vi "test Find and Initialize SLSC Switch CD.vi"(8 "error in (no error)":errorcluster, 11 "TestCase in":refnum<class "SLSC Switch Scripting Unit Tests.lvclass">) -> (0 "error out":errorcluster, 3 "TestCase out":refnum<class "SLSC Switch Scripting Unit Tests.lvclass">)   [LabVIEW 2017, in "SLSC Switch Scripting Unit Tests.lvclass"]
uses:
  SLSC Switch Scripting Unit Tests.lvclass
  C:/Program Files (x86)/National Instruments/LabVIEW 2017/vi.lib/addons/_JKI Toolkits/VI Tester/TestCase.llb/TestCase.lvclass
  <vilib>/addons/_JKI Toolkits/VI Tester/TestCase.llb/TestCase.lvclass
panel:
  in  "Save?":bool
  out "Output Filename":string
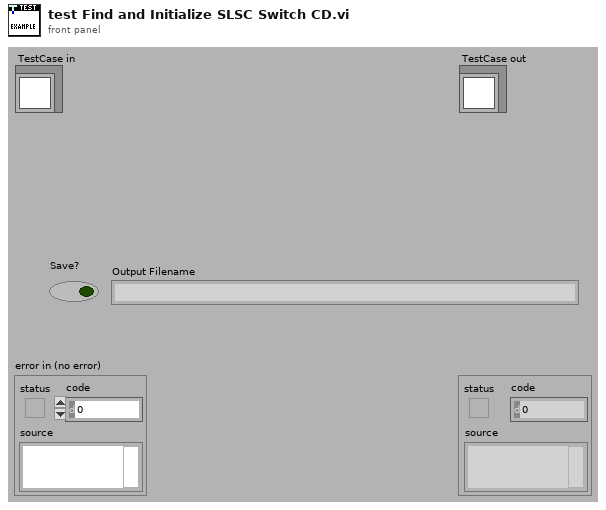
[diagram p1: front panel]
types:
  T1 = typedef "Custom Device API.lvlib/Custom Device Item Ref.ctl" = u64
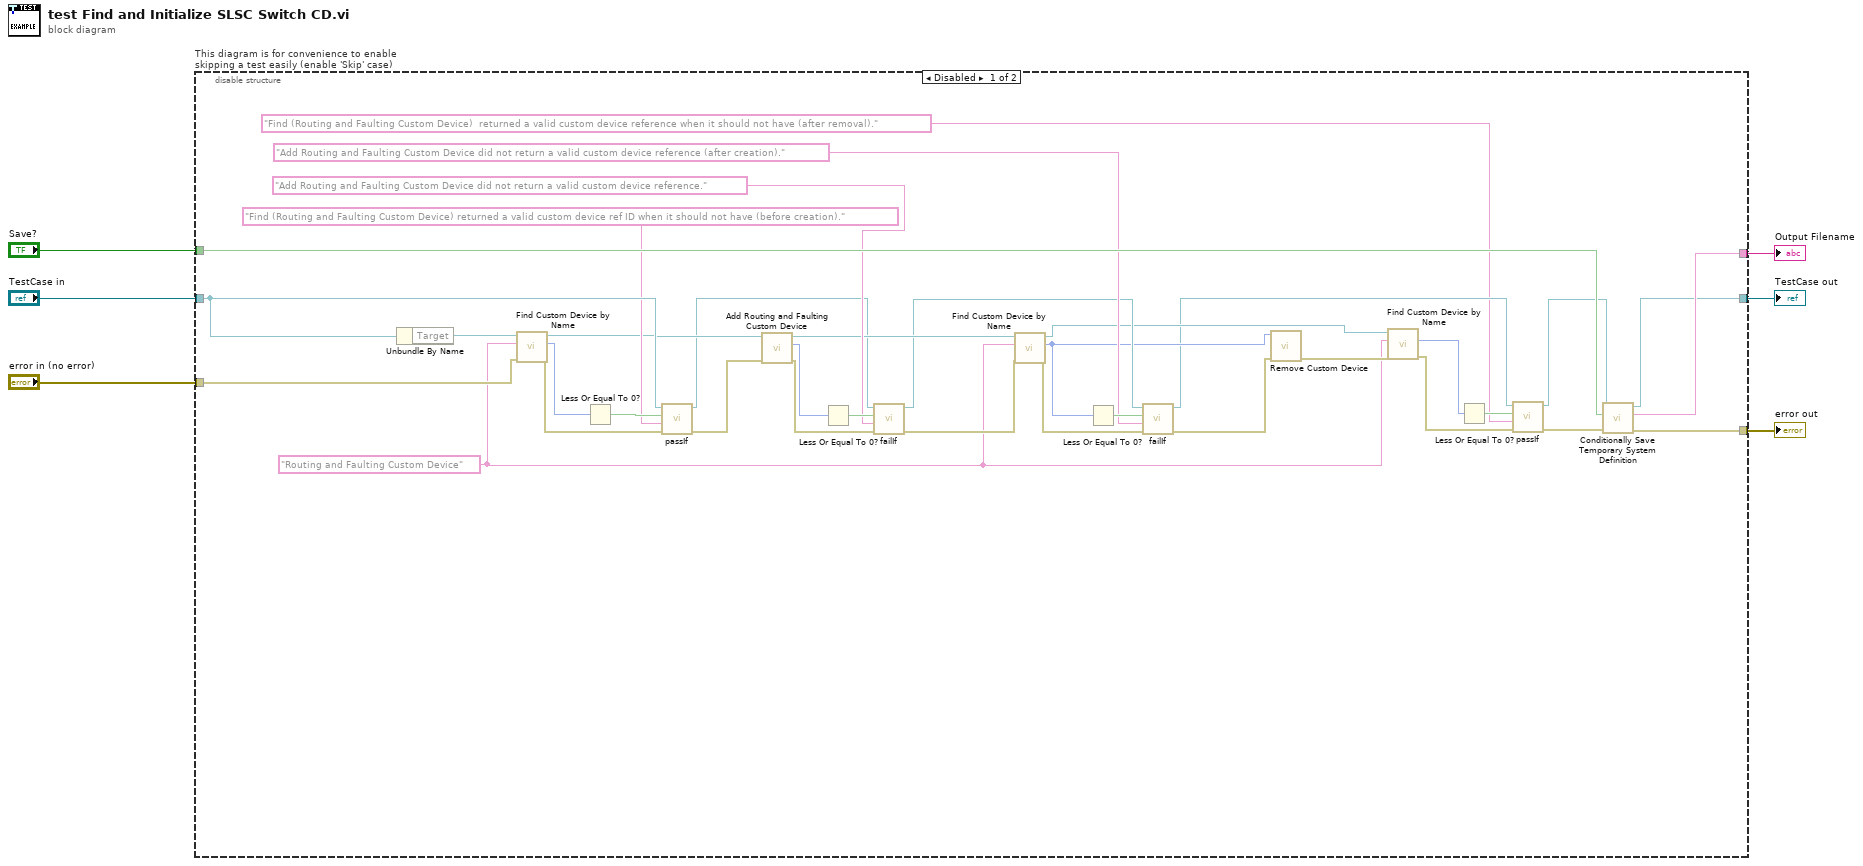
[diagram p0: block diagram]
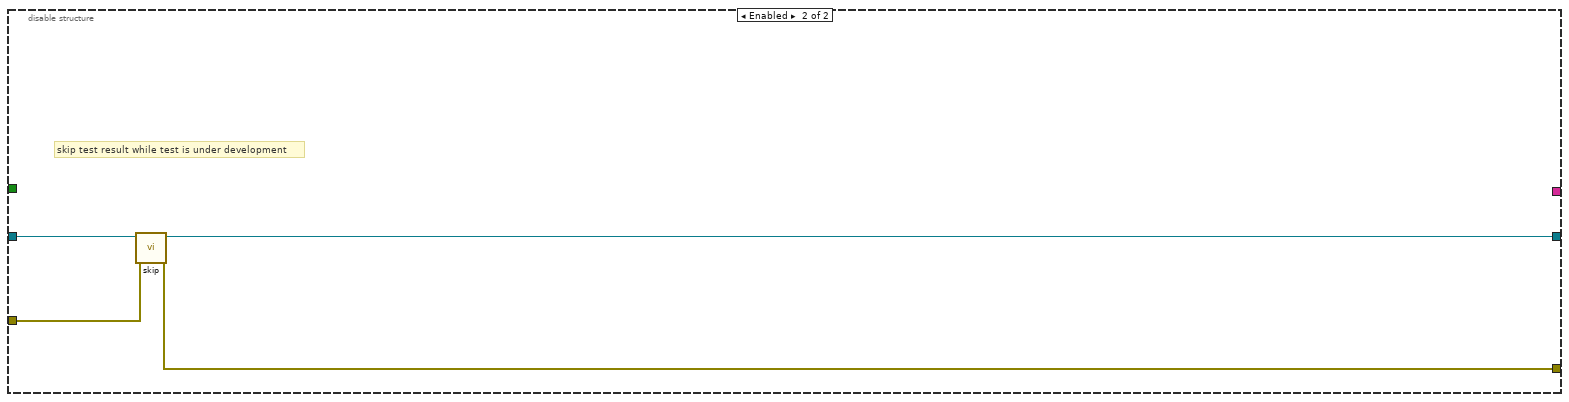
[diagram p2: hidden frame]
diagram:
  n1 = disable-structure "This diagram is for convenience to enable skipping a test easily (enable 'Skip' case)" shown="Disabled" {
    disable-tunnel: "TestCase in" -> [w36 w46]
    disable-tunnel: [w40 w44] -> w3
    disable-tunnel: [w41 w45] -> w5
    disable-tunnel: "error in (no error)" -> [w35 w43]
    disable-tunnel: [w42 _] -> w2
    disable-tunnel: "Save?" -> [w33 _]
    frame Disabled {
      w15 = "Routing and Faulting Custom Device" ("Name")
      n2 = Unbundle By Name(w36) -> ("Target"=w39:refnum<k24>)
      n3 = call "Find Custom Device by Name.vi"("error in (no error)"=w35, "Name"=w15, "Target in"=w39) -> ("error out"=w34:errorcluster, "CD Ref"=w38:T1, "Target out"=w31:refnum<k24>)  [unwired: 6 in]
      n4 = Less Or Equal To 0?(x=w38) -> (x <= 0?=w37:bool)
      n5 = call-dynamic "passIf.vi"("error in (no error)"=w34, "message (\"\")"="Find (Routing and Faulting Custom Device) returned a valid custom device ref ID when it should not have (before creation)." ("message (\"\")"), "pass"=w37, "TestCase in"=w36) -> ("error out"=w30:errorcluster, "TestCase out"=w21:refnum<class "SLSC Switch Scripting Unit Tests.lvclass">)  [unwired: 6 in]
      n6 = call "Add Routing and Faulting Custom Device.vi"("error in (no error)"=w30, "Target in"=w31) -> ("error out"=w27:errorcluster, "RaF CD Ref"=w29:T1, "Target out"=w25:refnum<k24>)  [unwired: 5 in, 2 out]
      n7 = Less Or Equal To 0?(x=w29) -> (x <= 0?=w28:bool)
      n8 = call-dynamic "failIf.vi"("error in (no error)"=w27, "message (\"\")"="Add Routing and Faulting Custom Device did not return a valid custom device reference." ("message (\"\")"), "fail"=w28, "TestCase in"=w21) -> ("error out"=w24:errorcluster, "TestCase out"=w20:refnum<class "SLSC Switch Scripting Unit Tests.lvclass">)  [unwired: 6 in]
      n9 = call "Find Custom Device by Name.vi"("error in (no error)"=w24, "Name"=w15, "Target in"=w25) -> ("error out"=w18:errorcluster, "CD Ref"=w19:T1, "Target out"=w17:refnum<k24>)  [unwired: 6 in]
      n10 = Less Or Equal To 0?(x=w19) -> (x <= 0?=w23:bool)
      n11 = call-dynamic "failIf.vi"("error in (no error)"=w18, "message (\"\")"="Add Routing and Faulting Custom Device did not return a valid custom device reference (after creation)." ("message (\"\")"), "fail"=w23, "TestCase in"=w20) -> ("error out"=w7:errorcluster, "TestCase out"=w12:refnum<class "SLSC Switch Scripting Unit Tests.lvclass">)  [unwired: 6 in]
      n12 = call "Remove Custom Device.vi"("error in (no error)"=w7, "RaF CD Ref"=w19) -> ("error out"=w16:errorcluster)  [unwired: 9 in]
      n13 = call "Find Custom Device by Name.vi"("error in (no error)"=w16, "Name"=w15, "Target in"=w17) -> ("error out"=w13:errorcluster, "CD Ref"=w10:T1)  [unwired: 6 in, 1 out]
      n14 = Less Or Equal To 0?(x=w10) -> (x <= 0?=w14:bool)
      n15 = call-dynamic "passIf.vi"("error in (no error)"=w13, "message (\"\")"="Find (Routing and Faulting Custom Device)  returned a valid custom device reference when it should not have (after removal)." ("message (\"\")"), "pass"=w14, "TestCase in"=w12) -> ("error out"=w8:errorcluster, "TestCase out"=w11:refnum<class "SLSC Switch Scripting Unit Tests.lvclass">)  [unwired: 6 in]
      n16 = call "Conditionally Save Temporary System Definition.vi"("error in (no error)"=w8, "Save?"=w33, "Test Case"=w11) -> ("error out"=w41:errorcluster, "filename"=w42:string, "Test Case"=w40:refnum<class "SLSC Switch Scripting Unit Tests.lvclass">)  [unwired: 6 in]
    }
    frame Enabled {
      # "skip test result while test is under development"
      n17 = call <vilib>:"skip.vi"("error in (no error)"=w43, "TestCase in"=w46) -> ("error out"=w45:errorcluster, "TestCase out"=w44:refnum<class "SLSC Switch Scripting Unit Tests.lvclass">)  [unwired: 8 in]
    }
  }
  "error out" <- w5
  "TestCase out" <- w3
  "Output Filename" <- w2
